vi "PQresultErrorField.vi"(7 "error in (no error)":errorcluster, 8 "fieldcode":T1(ring), 9 "res":u32) -> (0 "error out":errorcluster, 1 "resulterrorfield":string, 2 "res_out":u32)   [LabVIEW 2019, in "libpqlv.lvlib"]
doc: "Returns an individual field of an error report.\nThe client is responsible for formatting displayed information to meet its needs; in particular it should break long lines as needed. Newline characters appearing in the error message fields should be treated as paragraph breaks, not line breaks.\n\nErrors generated internally by libpq will have severity and primary message, but typically no other fields. Errors returned by a pre-3.0-protocol server will include severity and primary message, and sometimes a detail message, but no other fields.\n\nNote that error fields are only available from PGresult objects, not PGconn objects; there is no PQerrorField function.\nhttp://www.postgresql.org/docs/8.1/interactive/libpq-exec.html"
uses:
  libpqlv.lvlib
  libpq.dll
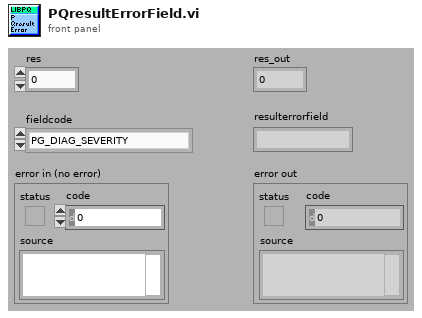
[diagram p1: front panel]
types:
  T1 = enum32{"PG_DIAG_SEVERITY", "PG_DIAG_SQLSTATE", "PG_DIAG_MESSAGE_PRIMARY", "PG_DIAG_MESSAGE_DETAIL", "PG_DIAG_MESSAGE_HINT", "PG_DIAG_STATEMENT_POSITION", "PG_DIAG_INTERNAL_POSITION", "PG_DIAG_INTERNAL_QUERY", "PG_DIAG_CONTEXT", "PG_DIAG_SOURCE_FILE", "PG_DIAG_SOURCE_LINE", "PG_DIAG_SOURCE_FUNCTION"}
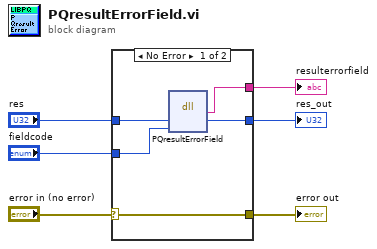
[diagram p0: block diagram]
diagram:
  n1 = case shown="No Error" "error in (no error)" {
    selector: "error in (no error)" -> [w11 w13]
    tunnel: [w11 w13] -> w5
    tunnel: [w10 _] -> w4
    tunnel: "fieldcode" -> [w9 _]
    tunnel: "res" -> [w8 w12]
    tunnel: [w7 w12] -> w2
    frame No Error {
      n2 = dll-call lib="libpq.*" fn="PQresultErrorField"("res"=w8, "fieldcode"=w9) -> ("resulterrorfield"=w10:string, "res"=w7:u32)  [unwired: 4 in, 2 out]
    }
    frame Error {
    }
  }
  "resulterrorfield" <- w4
  "error out" <- w5
  "res_out" <- w2
